vi "TxData_Organization_01.vi"() -> ()   [LabVIEW 2023, in "ParsingData.lvlib"]
uses:
  <vilib>/Utility/file.llb/Read Delimited Spreadsheet (DBL).vi
  ParsingData.lvlib
panel:
  in  "Input power_up":dbl
  in  "Input power_low":dbl
  out "EVM to EIRP":cluster{dbl[], "all rows":dbl[]}[](graph)
  out "all rows":dbl[][](array[numeric])
  out "filenames":string[](array[string])
  in  "path":path
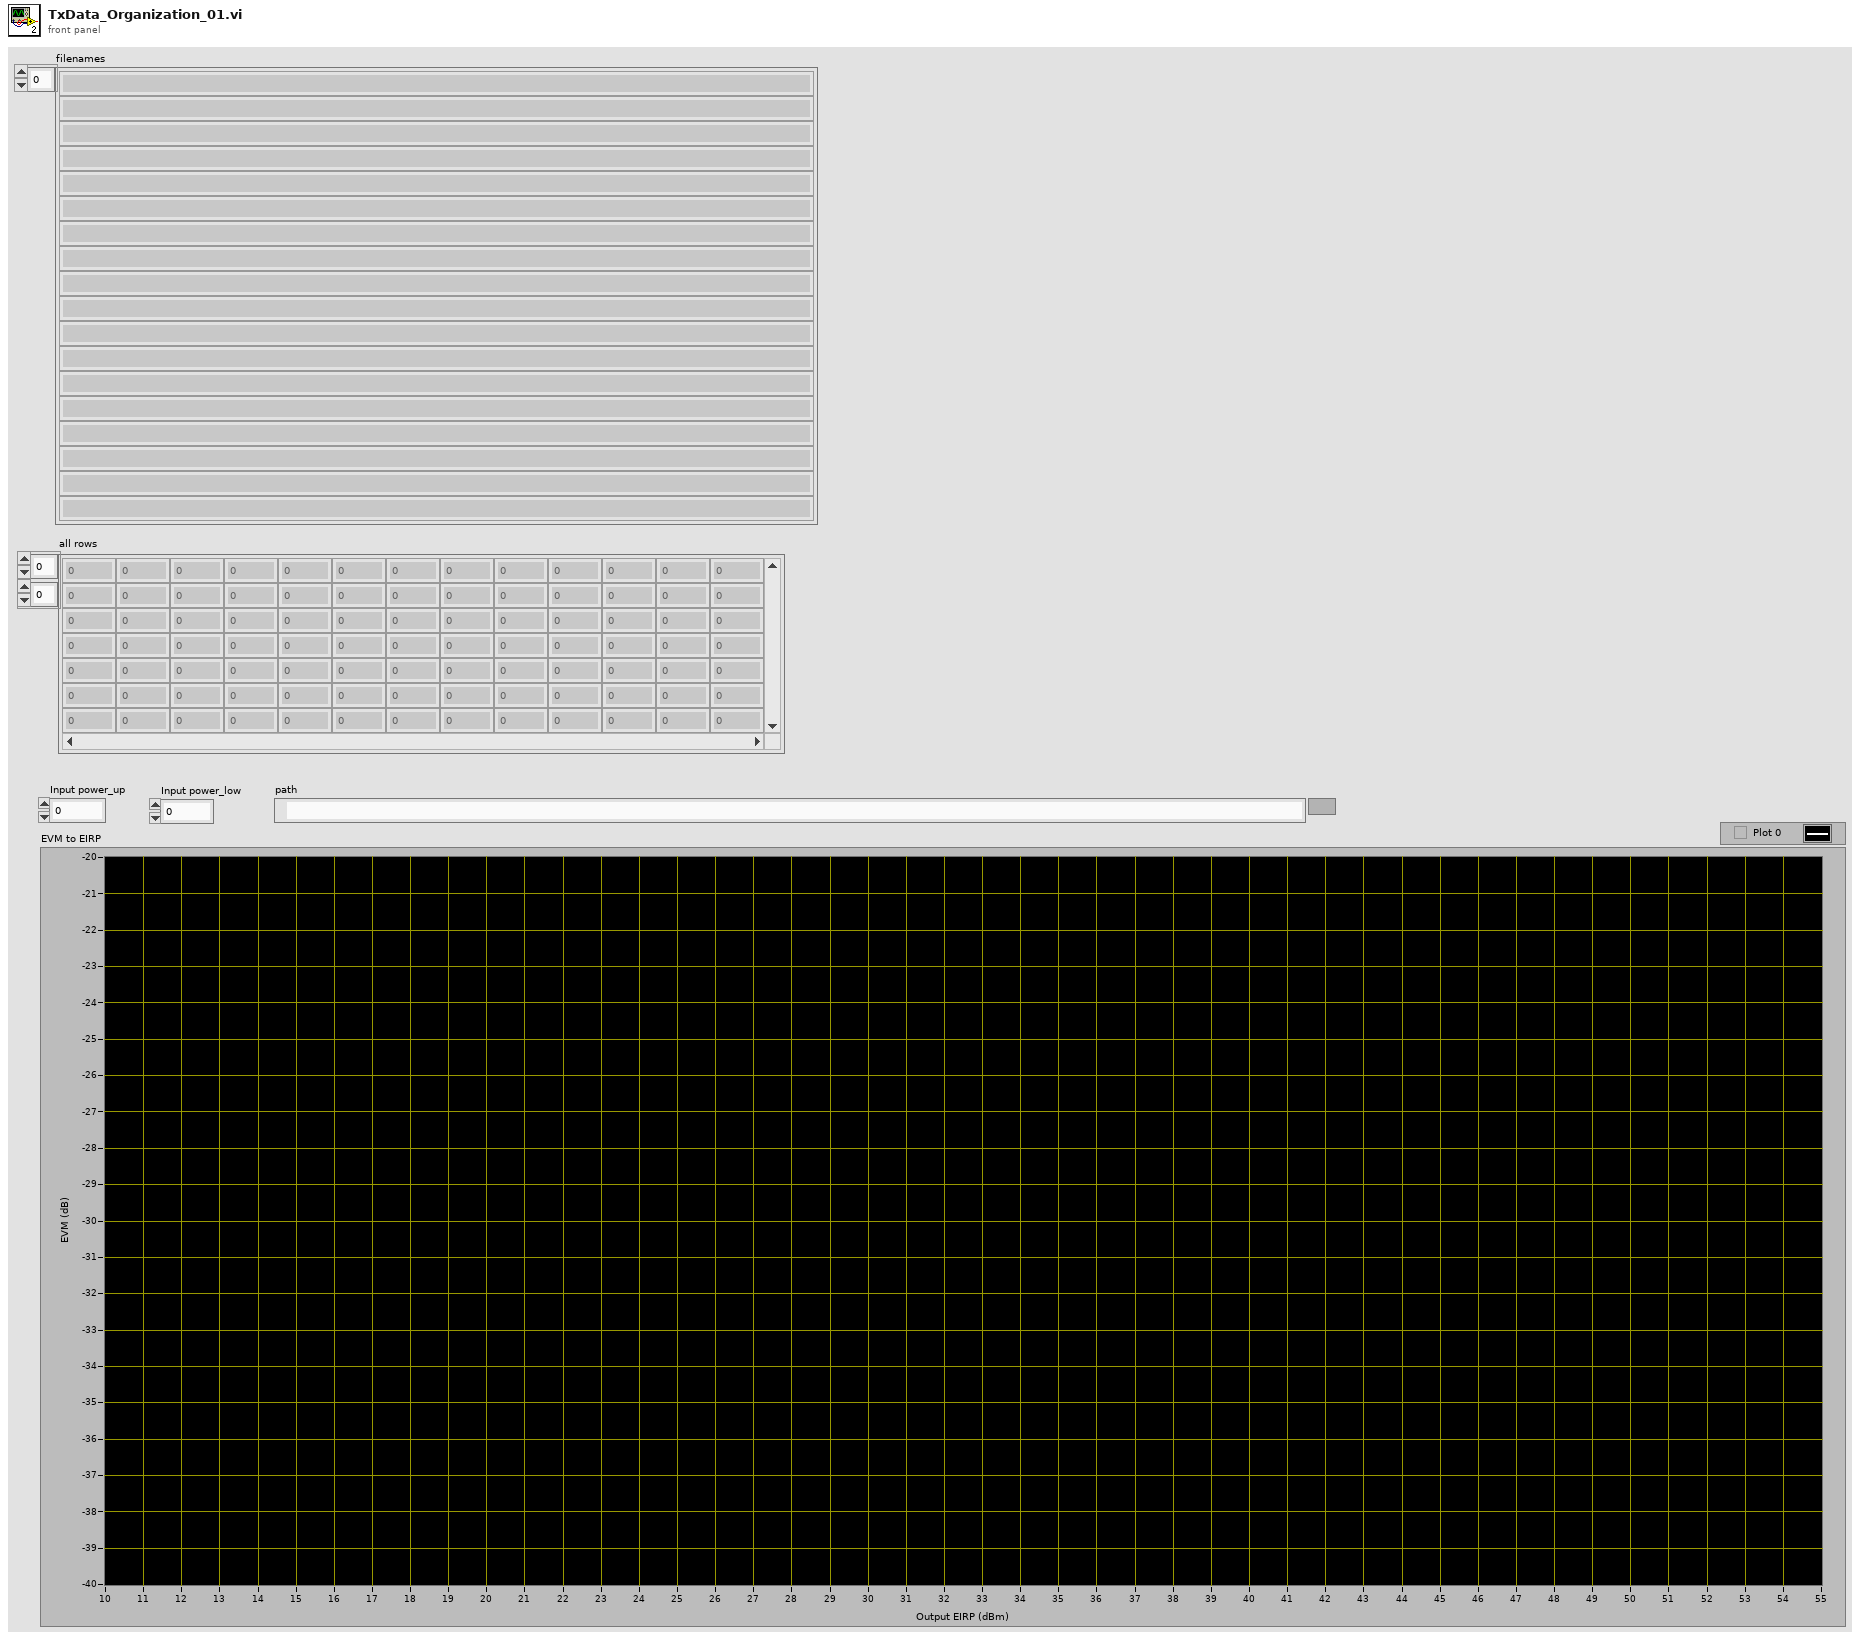
[diagram p1: front panel]
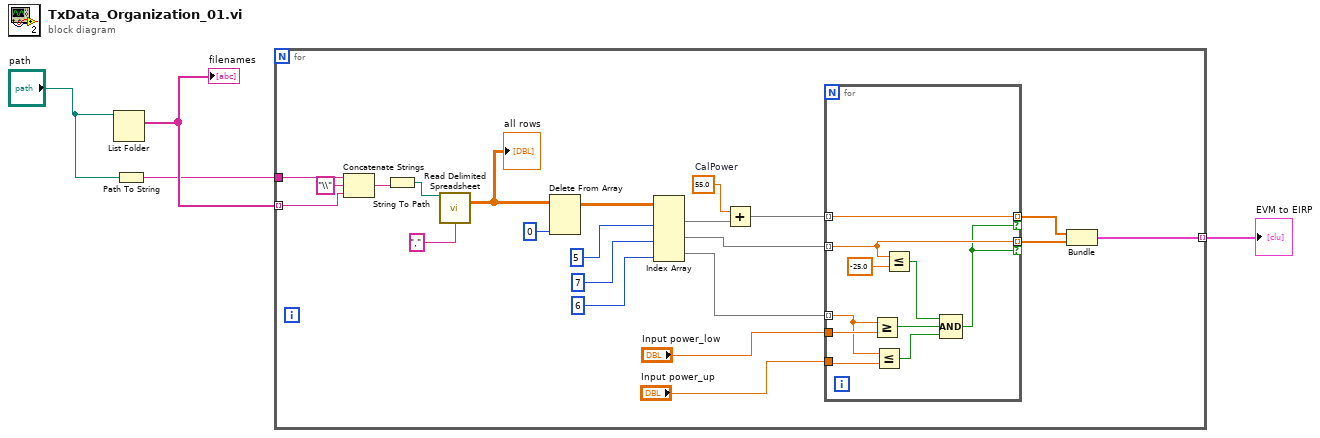
[diagram p0: block diagram]
diagram:
  n1 = List Folder(path="path") -> (filenames=w4:string[])  [unwired: 3 in, 3 out]
  "filenames" <- w4
  n2 = Path To String(path="path") -> (string=w2:string)
  n3 = for {
    tunnel: w4 -> [w22] mode=indexing
    tunnel: w2 -> [w26]
    tunnel: [w13] -> w1 mode=indexing
    w14 = 55.0  # CalPower
    n4 = Concatenate Strings(w26, "\\" ("string"), w22) -> (w25:string)
    n5 = String To Path(string=w25) -> (path=w24:path)
    n6 = call-poly <vilib>:"Read Delimited Spreadsheet.vi"("file path (dialog if empty)"=w24, "delimiter (\\t)"="," ("delimiter (\\t)")) -> ("all rows"=w20:dbl[][])  [unwired: 8 in, 5 out]
    "all rows" <- w20
    n7 = Delete From Array(array=w20, index (row)=0 ("disabled index (col)")) -> (array with subset deleted=w18:dbl[][])  [unwired: 2 in, 1 out]
    n8 = Index Array(array=w18, index (col) #1=5 ("disabled index (col)"), index (col) #2=7 ("index (col)"), index (col) #3=6 ("index (col)")) -> (element #1=w15:dbl[], element #2=w11:dbl[], element #3=w7:dbl[])  [unwired: 3 in]
    n9 = Add(x=w14, y=w15) -> (x+y=w12:dbl[])
    n10 = for {
      tunnel: w12 -> [w34] mode=indexing
      tunnel: w11 -> [w35] mode=indexing
      tunnel: [w35] -> w9 mode=indexing if=w27
      tunnel: [w34] -> w10 mode=indexing if=w27
      tunnel: w7 -> [w32] mode=indexing
      tunnel: "Input power_low" -> [w33]
      tunnel: "Input power_up" -> [w31]
      n11 = Greater Or Equal?(x=w32, y=w33) -> (x >= y?=w29:bool)
      n12 = Less Or Equal?(x=w32, y=w31) -> (x <= y?=w30:bool)
      n13 = Less Or Equal?(x=w35, y=-25.0) -> (x <= y?=w28:bool)
      n14 = Compound Arithmetic op=AND(w28, w29, w30) -> (w27:bool)
    }
    n15 = Bundle(w10, w9) -> (w13:cluster{dbl[], dbl[]})  [unwired: 1 in]
  }
  "EVM to EIRP" <- w1
